vi "LOG_sim_2 (SubVI).vi"(4 "Rotation":T5, 5 "Time":T1, 6 "act_b":T6, 7 "Position":T4, 9 "Aerodyn":T2, 10 "M_alpha [rad/s^2], M_beta [rad/s^2]":T3, 11 "acc [m/s^2]":dbl[](array[numeric])) -> ()   [LabVIEW 2017]
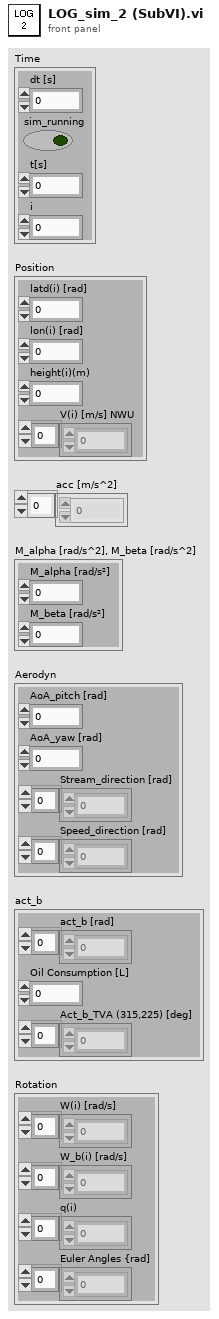
[diagram p1: front panel]
types:
  T1 = cluster{"dt [s]":dbl, "sim_running":bool, "t[s]":dbl, "i":i32}
  T2 = cluster{"AoA_pitch [rad]":dbl, "AoA_yaw [rad]":dbl, "Stream_direction [rad]":dbl[], "Speed_direction [rad]":dbl[]}
  T3 = cluster{"M_alpha [rad/s²]":dbl, "M_beta [rad/s²]":dbl}
  T4 = cluster{"latd(i) [rad]":dbl, "lon(i) [rad]":dbl, "height(i)(m)":dbl, "V(i) [m/s] NWU":dbl[]}
  T5 = cluster{"W(i) [rad/s]":dbl[], "W_b(i) [rad/s]":dbl[], "q(i)":dbl[], "Euler Angles {rad]":dbl[]}
  T6 = cluster{"act_b [rad]":dbl[], "Oil Consumption [L]":dbl, "Act_b_TVA (315,225) [deg]":dbl[]}
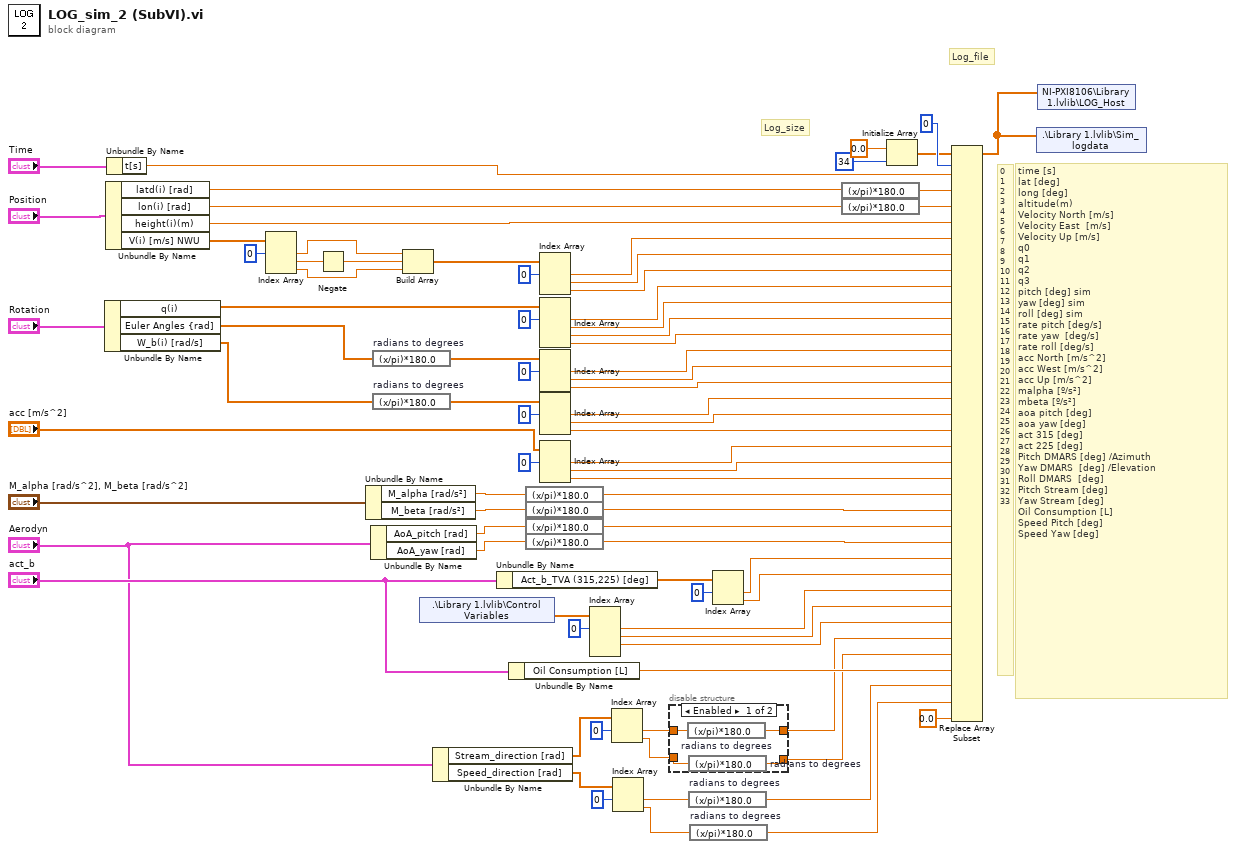
[diagram p0: block diagram]
diagram:
  # "Log_file"
  # "Log_size"
  # "0\n1\n2\n3\n4\n5\n6\n7\n8\n9\n10\n11\n12\n13\n14\n15\n16\n17\n18\n19\n20\n21\n22\n23\n24\n25\n26\n27\n28\n29\n30\n31\n32\n33"
  # "time [s]\nlat [deg]\nlong [deg]\naltitude(m)\nVelocity North [m/s]\nVelocity East  [m/s]\nVelocity Up [m/s]\nq0\nq1\nq2\nq3\npitch [deg] sim\nyaw [deg] sim\nroll [deg] sim\nrate pitch [deg/s] \nrate yaw  [deg/s]\nrate roll [deg/s]\nacc North [m/s^2] \nacc West [m/s^2]\nacc Up [m/s^2]\nmalpha [º/s²]\nmbeta [º/s²]\naoa pitch [deg] \naoa yaw [deg]\nact 315 [deg] \nact 225 [deg]\nPitch DMARS [deg] /Azimuth\nYaw DMARS  [deg] /Elevation\nRoll DMARS  [deg]\nPitch Stream [deg]\nYaw Stream [deg]\nOil Consumption [L]\nSpeed Pitch [deg]\nSpeed Yaw [deg]"
  n1 = Unbundle By Name("Rotation") -> ("q(i)"=w78:dbl[], "Euler Angles {rad]"=w2:dbl[], "W_b(i) [rad/s]"=w1:dbl[])
  n2 = Unbundle By Name("Position") -> ("latd(i) [rad]"=w73:dbl, "lon(i) [rad]"=w74:dbl, "height(i)(m)"=w75:dbl, "V(i) [m/s] NWU"=w76:dbl[])
  n3 = Unbundle By Name("Time") -> ("t[s]"=w67:dbl)
  n4 = Index Array(array=w76, index #1=0 ("index")) -> (element #1=w39:dbl, element #2=w37:dbl, element #3=w40:dbl)  [unwired: 2 in]
  n5 = Negate(x=w37) -> (-x=w38:dbl)
  n6 = Unbundle By Name("M_alpha [rad/s^2], M_beta [rad/s^2]") -> ("M_alpha [rad/s²]"=w57:dbl, "M_beta [rad/s²]"=w58:dbl)
  n7 = Unbundle By Name("Aerodyn") -> ("AoA_pitch [rad]"=w59:dbl, "AoA_yaw [rad]"=w60:dbl)
  n8 = expression code="(x/pi)*180.0" "radians to degrees"(w2) -> (w61:dbl[])
  n9 = expression code="(x/pi)*180.0" "radians to degrees"(w1) -> (w23:dbl[])
  n10 = Build Array(w39, w38, w40) -> (w79:dbl[])
  n11 = shared-variable ".\\Library 1.lvlib\\Control Variables"() -> (w63:dbl[])  [unwired: 1 in, 1 out]
  n12 = Unbundle By Name("Aerodyn") -> ("Stream_direction [rad]"=w62:dbl[], "Speed_direction [rad]"=w69:dbl[])
  n13 = Unbundle By Name("act_b") -> ("Act_b_TVA (315,225) [deg]"=w80:dbl[])
  n14 = Unbundle By Name("act_b") -> ("Oil Consumption [L]"=w82:dbl)
  n15 = expression code="(x/pi)*180.0" ("radians to degrees")(w57) -> (w32:dbl)
  n16 = expression code="(x/pi)*180.0" ("radians to degrees")(w58) -> (w33:dbl)
  n17 = expression code="(x/pi)*180.0" ("radians to degrees")(w59) -> (w44:dbl)
  n18 = expression code="(x/pi)*180.0" ("radians to degrees")(w60) -> (w45:dbl)
  n19 = Index Array(array=w79, index #1=0 ("index")) -> (element #1=w11:dbl, element #2=w12:dbl, element #3=w13:dbl)  [unwired: 2 in]
  n20 = Index Array(array=w78, index #1=0 ("index")) -> (element #1=w15:dbl, element #2=w16:dbl, element #3=w17:dbl, element #4=w18:dbl)  [unwired: 3 in]
  n21 = Index Array(array=w61, index #1=0 ("index")) -> (element #1=w19:dbl, element #2=w20:dbl, element #3=w21:dbl)  [unwired: 2 in]
  n22 = Index Array(array=w23, index #1=0 ("index")) -> (element #1=w24:dbl, element #2=w25:dbl, element #3=w26:dbl)  [unwired: 2 in]
  n23 = Index Array(array="acc [m/s^2]", index #1=0 ("index")) -> (element #1=w28:dbl, element #2=w29:dbl, element #3=w30:dbl)  [unwired: 2 in]
  n24 = Index Array(array=w63, index #1=0 ("index")) -> (element #1=w55:dbl, element #2=w56:dbl, element #3=w54:dbl)  [unwired: 3 in, 1 out]
  n25 = Index Array(array=w62, index #1=0 ("index")) -> (element #1=w41:dbl, element #2=w43:dbl)  [unwired: 1 in]
  n26 = Index Array(array=w69, index #1=0 ("index")) -> (element #1=w50:dbl, element #2=w48:dbl)  [unwired: 1 in]
  n27 = disable-structure shown="Enabled" {
    disable-tunnel: w41 -> [w86 w88]
    disable-tunnel: w43 -> [w85 w87]
    disable-tunnel: [w84 w88] -> w46
    disable-tunnel: [w83 w87] -> w47
    frame Enabled {
      n28 = expression code="(x/pi)*180.0" "radians to degrees"(w86) -> (w84:dbl)
      n29 = expression code="(x/pi)*180.0" "radians to degrees"(w85) -> (w83:dbl)
    }
    frame Disabled {
    }
  }
  n30 = expression code="(x/pi)*180.0" "radians to degrees"(w50) -> (w51:dbl)
  n31 = expression code="(x/pi)*180.0" "radians to degrees"(w48) -> (w52:dbl)
  n32 = Index Array(array=w80, index #1=0 ("index")) -> (element #1=w64:dbl, element #2=w65:dbl)  [unwired: 1 in]
  n33 = expression code="(x/pi)*180.0" ("radians to degrees")(w73) -> (w8:dbl)
  n34 = expression code="(x/pi)*180.0" ("radians to degrees")(w74) -> (w9:dbl)
  n35 = Initialize Array(0.0 ("element"), 34 ("dimension size")) -> (w5:dbl[])
  n36 = Replace Array Subset(array=w5, new element #1=w67, index #1=0 ("index"), new element #2=w8, new element #3=w9, new element #4=w75, new element #5=w11, new element #6=w12, new element #7=w13, new element #8=w15, new element #9=w16, new element #10=w17, new element #11=w18, new element #12=w19, new element #13=w20, new element #14=w21, new element #15=w24, new element #16=w25, new element #17=w26, new element #18=w28, new element #19=w29, new element #20=w30, new element #21=w32, new element #22=w33, new element #23=w44, new element #24=w45, new element #25=w64, new element #26=w65, new element #27=w55, new element #28=w56, new element #29=w54, new element #30=w46, new element #31=w47, new element #32=w82, new element #33=w51, new element #34=w52, new element #35=0.0 ("new element/subarray")) -> (w35:dbl[])  [unwired: 34 in]
  n37 = shared-variable ".\\Library 1.lvlib\\Sim_logdata"(w35) -> ()  [unwired: 1 in, 1 out]
  n38 = shared-variable "NI-PXI8106\\Library 1.lvlib\\LOG_Host"(w35) -> ()  [unwired: 1 in, 1 out]
